vi "Emballage_BDD_CreationRapportParCarton.vi"(8 "error in (no error)":errorcluster caption="entrée d'erreur (pas d'erreur)", 10 "Tableau n° valves":string[](array[string]), 11 "N° Cmd":string) -> (0 "error out":errorcluster caption="sortie d'erreur", 1 "fichier erroné":bool, 2 "chemin complet":path, 3 "chaîne concaténée":string)   [LabVIEW 2020]
doc: "Envoi un mail avec la liste des valves emballées en pièce jointe si spécifié dans le fichier XML PP de la valve (FlatProp) ou correspondance produit code barre.txt (autres valves)"
uses:
  Modules/FS/60_FS_Controles/60_FS_SetGet.ctl
panel:
  out "temps Exe [s]":dbl
  out "Liste n° pièces de la cmde":string[](array[string])
  out "Carton":string[](array[string])
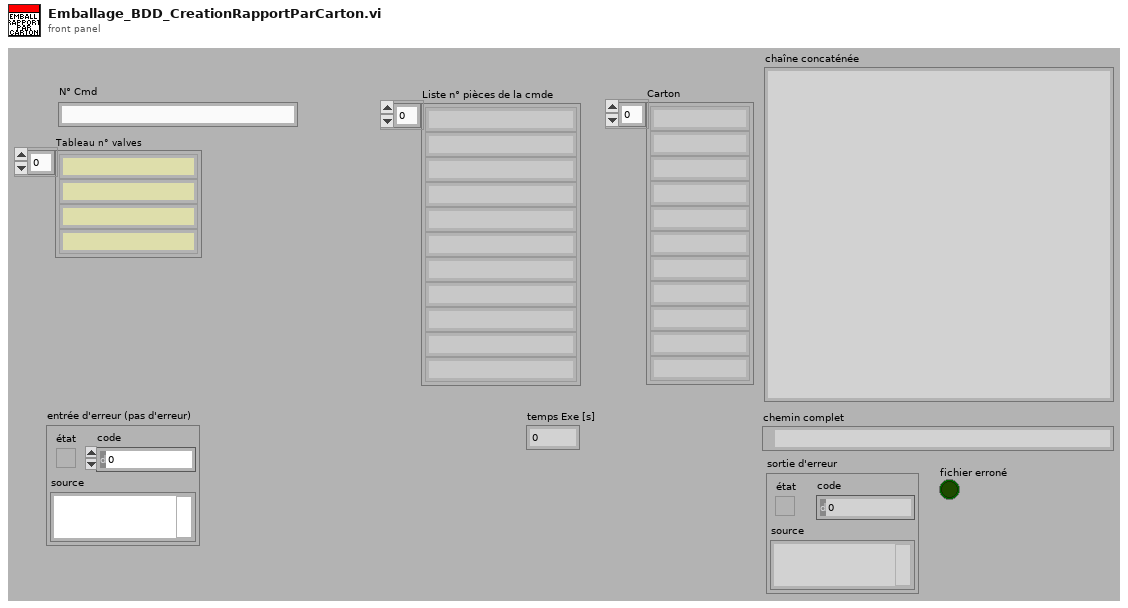
[diagram p1: front panel]
types:
  T1 = typedef "60_FS_SetGet.ctl" = enum16{"set", "get"}
  T2 = enum16{"open", "replace", "create", "open or create", "replace or create", "replace or create with confirmation"}
  T3 = typedef "DATA commande.ctl" = cluster{"n°article FAS":string, "n° cmde FAS":string, "quantité cmde":string, "ID LIG cmde":string, "n° cmde client":string, "nom client":string, "n° article client":string, "indice revision client":string, "société de facturation":string, "langue a utiliser":string}
  T4 = cluster{"Admin-réseau":path, "XML-Réseau":path, " Résultat tests-Réseau":path, " Archive prôbleme-Réseau":path, " Archive Test  Local":path}
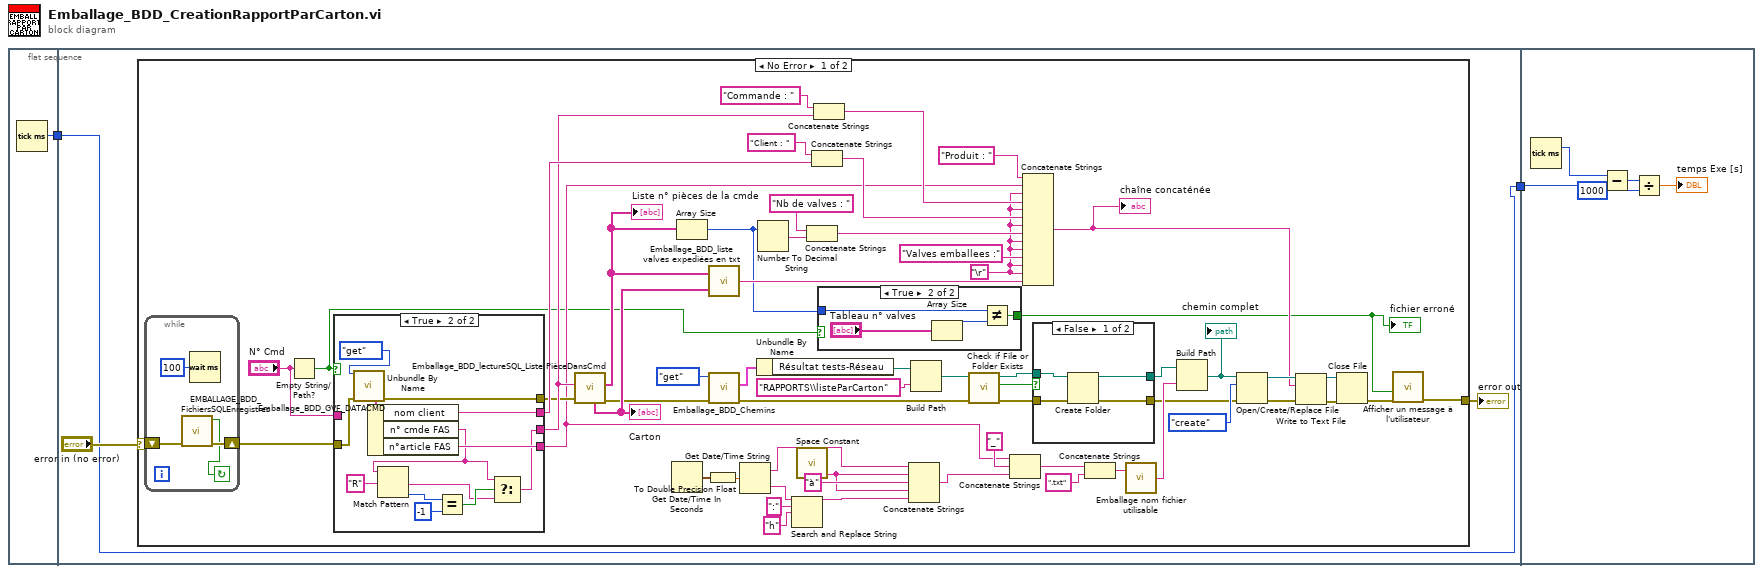
[diagram p0: block diagram]
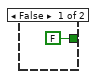
[diagram p2: hidden frame]
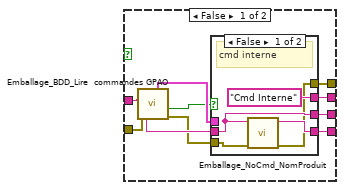
[diagram p3: hidden frame]
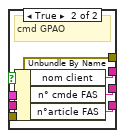
[diagram p4: hidden frame]
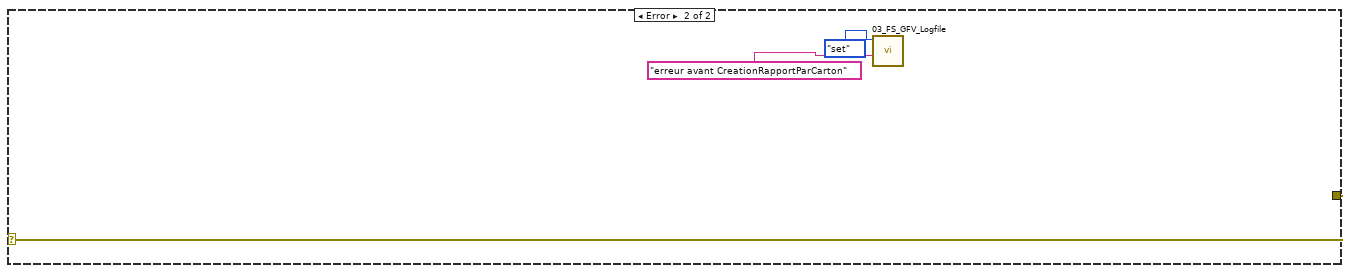
[diagram p6: hidden frame]
diagram:
  n1 = flat-sequence {
    tunnel: [w3] -> w2
    tunnel: w2 -> [w4]
    tunnel: [w4] -> w1
    tunnel: w1 -> [w116]
    frame #0 {
      n2 = Tick Count (ms)() -> (millisecond timer value=w3:u32)
    }
    frame #1 {
      n3 = case shown="No Error" "error in (no error)" {
        selector: "error in (no error)" -> [w13 w115]
        tunnel: [w10 w115] -> w5
        frame No Error {
          w56 = "\r"
          n4 = while {
            shift-right: [w73] -> w12
            shift-left: w13 -> [w74]
            stop <- w72 continue-if-true
            n5 = call "EMBALLAGE_BDD_FichiersSQLEnregistres.vi"("Error in"=w74) -> ("Error out"=w73:errorcluster, "Dans la gamme ?"=w72:bool)  [unwired: 9 in]
            n6 = Wait (ms)(milliseconds to wait=u32 100 ("attente (ms)")) -> ()  [unwired: 1 out]
          }
          n7 = Empty String/Path?(string/path="N° Cmd") -> (empty?=w7:bool)
          n8 = case shown="True" w7 {
            tunnel: w12 -> [w83 w104]
            tunnel: [w75 w103] -> w16
            tunnel: [w80 w96] -> w14
            tunnel: [w82 w102] -> w22
            tunnel: [w81 w94] -> w21
            tunnel: "N° Cmd" -> [w77 _]
            frame False {
              n9 = call "Emballage_BDD_Lire  commandes GPAO.vi"("error in"=w83, "Numéro commande"=w77) -> ("error out"=w76:errorcluster, "existe ?"=w78:bool, "DATA cmde"=w79:T3)  [unwired: 4 in, 3 out]
              n10 = case shown="False" w78 {
                tunnel: ["Cmd Interne" ("nom client") w93] -> w82
                tunnel: [w87 w92] -> w81
                tunnel: [w86 w91] -> w80
                tunnel: w79 -> [_ w90]
                tunnel: w77 -> [w87 _]
                tunnel: w76 -> [w85 w89]
                tunnel: [w84 w89] -> w75
                frame False {
                  # "cmd interne"
                  n11 = call "Emballage_NoCmd_NomProduit.vi"("Error in"=w85, "NO_CDEVAL"=w87) -> ("Error out"=w84:errorcluster, "Produit"=w86:string)  [unwired: 8 in]
                }
                frame True {
                  # "cmd GPAO"
                  n12 = Unbundle By Name(w90) -> ("nom client"=w93:string, "n° cmde FAS"=w92:string, "n°article FAS"=w91:string)
                }
              }
            }
            frame True {
              n13 = call "Emballage_BDD_GVF_DATACMD.vi"("SetGet"=60_FS_SetGet."get", "Error in"=w104) -> ("DATA cmde OUT"=w105:T3, "Error out"=w103:errorcluster)  [unwired: 6 in, 6 out]
              n14 = Unbundle By Name(w105) -> ("nom client"=w102:string, "n° cmde FAS"=w95:string, "n°article FAS"=w96:string)
              n15 = Match Pattern(string=w95, regular expression="R" ("expression régulière")) -> (after substring=w99:string, offset past match=w100:i32)  [unwired: 1 in, 2 out]
              n16 = Equal?(x=w100, y=-1) -> (x = y?=w101:bool)
              n17 = Select(t=w95, s=w101, f=w99) -> (s? t:f=w94:string)
            }
          }
          n18 = call "Emballage_BDD_lectureSQL_Liste PièceDansCmd.vi"("Error in"=w16, "NO_CDEVAL"=w21) -> ("Error out"=w17:errorcluster, "Liste n° pièces de la cmde"=w24:string[], "Carton"=w25:string[])  [unwired: 5 in, 2 out]
          "Carton" <- w25
          "Liste n° pièces de la cmde" <- w24
          n19 = Get Date/Time In Seconds() -> (seconds since 1Jan1904=w53:timestamp)
          n20 = Array Size(array=w24) -> (size(s)=w8:i32)
          n21 = To Double Precision Float(number=w53) -> (double precision float=w54:dbl)
          n22 = call "Emballage_BDD_liste valves expediées en txt.vi"("Carton"=w25, "Liste n° pièces de la cmde"=w24) -> ("liste valves"=w26:string)
          n23 = call "Emballage_BDD_Chemins.vi"("error in (no error)"=w17, "SetGet"=60_FS_SetGet."get") -> ("error out"=w23:errorcluster, "CLT_Chemins_out"=w31:T4)  [unwired: 8 in]
          n24 = Get Date/Time String(seconds (now)=w54) -> (date string=w47:string, time string=w50:string)  [unwired: 2 in]
          n25 = Unbundle By Name(w31) -> ("Résultat tests-Réseau"=w30:path)
          n26 = Number To Decimal String(number=w8) -> (decimal integer string=w60:string)  [unwired: 1 in]
          n27 = Search and Replace String(input string=w50, search string=":" ("chaîne recherchée"), replace string="h" ("chaîne de remplacement (\"\")")) -> (result string=w48:string)  [unwired: 5 in, 3 out]
          n28 = call <vilib>:"Space Constant.vi"() -> ("String"=w46:string)
          n29 = Concatenate Strings("Nb de valves : " ("expression régulière"), w60) -> (w63:string)
          n30 = Concatenate Strings("Client : " ("expression régulière"), w22) -> (w57:string)
          n31 = Concatenate Strings("Commande : " ("expression régulière"), w21) -> (w64:string)
          n32 = case shown="True" w7 {
            tunnel: [FALSE w70] -> w9
            tunnel: w8 -> [_ w69]
            frame False {
            }
            frame True {
              n33 = Array Size(array="Tableau n° valves") -> (size(s)=w68:i32)
              n34 = Not Equal?(x=w69, y=w68) -> (x != y?=w70:bool)
            }
          }
          "fichier erroné" <- w9
          n35 = Concatenate Strings(w47, w46, "à" ("chaîne"), w46, w48) -> (w45:string)
          n36 = Build Path(base path=w30, name or relative path="RAPPORTS\\listeParCarton" ("chemin local RELEVES AUTOM\\EMBALL_...")) -> (appended path=w28:path)
          n37 = call <vilib>:"Check if File or Folder Exists.vi"("error in (no error)"=w23, "path"=w28) -> ("error out"=w34:errorcluster, "file or folder exists?"=w35:bool, "dup path"=w33:path)  [unwired: 7 in]
          n38 = Concatenate Strings(w14, "_", w45) -> (w20:string)
          n39 = Concatenate Strings("Produit : " ("expression régulière"), w14, w56, w64, w56, w57, w56, w63, w56, w56, "Valves emballees :" ("chaîne"), w56, w56, w26) -> (w37:string)
          "chaîne concaténée" <- w37
          n40 = case shown="False" w35 {
            tunnel: [w109 w112] -> w18
            tunnel: w34 -> [w110 w112]
            tunnel: w33 -> [w108 w111]
            tunnel: [w107 w111] -> w32
            frame False {
              n41 = Create Folder(path (use dialog)=w108, error in=w110) -> (created path=w107:path, error out=w109:errorcluster)  [unwired: 1 in, 1 out]
            }
            frame True {
            }
          }
          n42 = Concatenate Strings(w20, ".txt" ("chaîne")) -> (w44:string)
          n43 = call "Emballage nom fichier utilisable.vi"("chaîne en entrée"=w44) -> ("chaîne résultante"=w43:string)
          n44 = Build Path(base path=w32, name or relative path=w43) -> (appended path=w36:path)
          "chemin complet" <- w36
          n45 = Open/Create/Replace File(file path (use dialog)=w36, error in=w18, operation (0:open)=T2."create" ("opération (0 : open)")) -> (refnum out=w40:refnum<file>, error out=w38:errorcluster)  [unwired: 3 in, 1 out]
          n46 = Write to Text File(file (use dialog)=w40, text=w37, error in=w38) -> (refnum out=w42:refnum<file>, error out=w41:errorcluster)  [unwired: 1 in, 1 out]
          n47 = Close File(refnum=w42, error in=w41) -> (error out=w11:errorcluster)  [unwired: 1 out]
          n48 = call "Afficher un message à l'utilisateur"("error in (no error)"=w11, "Enable"=w9) -> ("error out"=w10:errorcluster)  [unwired: 8 in, 1 out]
        }
        frame Error {
          n49 = call "03_FS_GFV_Logfile.vi"("Chaîne"="erreur avant CreationRapportParCarton", "States"=60_FS_SetGet."set") -> ()  [unwired: 8 in, 2 out]
        }
      }
      "error out" <- w5
    }
    frame #2 {
      n50 = Tick Count (ms)() -> (millisecond timer value=w117:u32)
      n51 = Subtract(x=w117, y=w116) -> (x-y=w120:u32)
      n52 = Divide(x=w120, y=u32 1000) -> (x/y=→"temps Exe [s]":dbl)
    }
  }
